vi "项目路径.vi"() -> ()   [LabVIEW 2013]
panel:
  in  "项目路径":path
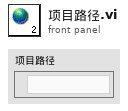
[diagram p1: front panel]
diagram:
